vi "Write G08 Specific.vi"(8 "error in (no error)":errorcluster, 9 "Done Signal":u32(ring)=16 format="%04x" items=["Local Primary"=1, "Local Secondary"=2, "Local Force"=4, "Master Primary"=16], 10 "Go Signal":u32(ring)=16 format="%04x" items=["Local Primary"=1, "Local Secondary"=2, "Local Force"=4, "Resynchronize"=8, "Master Primary"=16, "Master Secondary"=32, "Master Force"=64, "System Clock"=128, "Delay Clock"=256, "Inhibit Local"=512, "Start Local"=1024, "Start Bus"=2048, "Step Back Local"=4096, "Step Back Bus"=8192, "From E"=65536, "From F"=131072, "From Bus"=262144], 11 "BME_DG_G08_Chnl in":refnum<class "BME_DG_G05P2_Chnl.lvclass">) -> (0 "error out":errorcluster, 3 "BME_DG_G08_Chnl out":refnum<class "BME_DG_G05P2_Chnl.lvclass">)   [LabVIEW 2009, in "BME_DG_G05P2_Chnl.lvclass"]
uses:
  BME_DG_G05P2_Chnl.lvclass
  BME_DG_G05P2_Chnl.lvclass/BME_DG_G05P2_Chnl.ctl
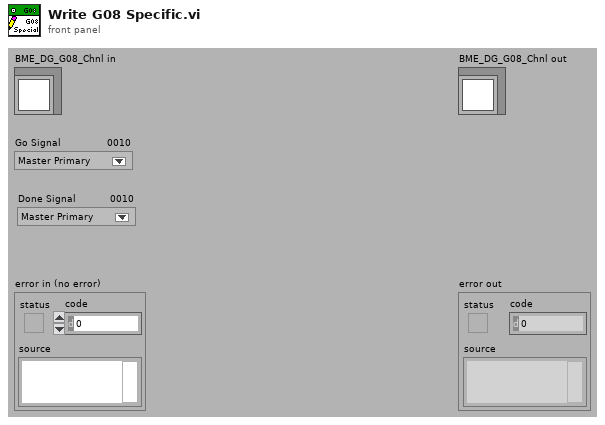
[diagram p1: front panel]
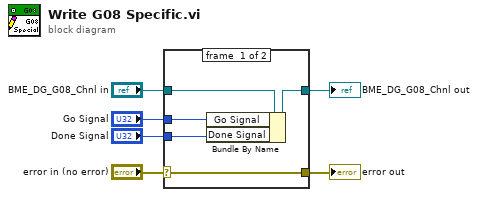
[diagram p0: block diagram]
diagram:
  n1 = case shown="No Error" "error in (no error)" {
    selector: "error in (no error)" -> [w11 w12]
    tunnel: [w11 w12] -> w5
    tunnel: [w9 w13] -> w3
    tunnel: "BME_DG_G08_Chnl in" -> [w10 w13]
    tunnel: "Go Signal" -> [w8 _]
    tunnel: "Done Signal" -> [w7 _]
    frame #0 {
      n2 = Bundle By Name(cluster=w10, "Go Signal"=w8, "Done Signal"=w7) -> (w9:refnum<class "BME_DG_G05P2_Chnl.lvclass">)
    }
    frame #1 {
    }
  }
  "error out" <- w5
  "BME_DG_G08_Chnl out" <- w3
